vi "BASE_Reporting.vi"(8 "error in (no error)":errorcluster) -> (0 "error out":errorcluster)   [LabVIEW 2017]
uses:
  <vilib>/Utility/miscctls.llb/LVRangeTypeDef.ctl
  <vilib>/Utility/miscctls.llb/LVRowAndColumnTypeDef.ctl
  <vilib>/Utility/miscctls.llb/LVRowAndColumnUnsignedTypeDef.ctl
  <vilib>/addons/database/Connection.llb/DB Tools Open Connec (Path).vi
  <vilib>/Utility/file.llb/Write Delimited Spreadsheet (string).vi
  <vilib>/addons/database/NI_Database_API.lvlib
panel:
  in  "Horizontal Slider Control":dbl(slide)=1.0 scale=0.0..19.0
  in  "Vertical Slider Control":dbl(slide)=1.0
  out "From Date":string
  out "appended path":path
  in  "SELECT FILTER":string(combo)="PART_NO"
  in  "Export to Excel":bool
  out "DESCRIPTION":string
  out "Data History Table":string[][](table)
  in  "TO DATE":timestamp format="%<%d/%m/%Y>T"
  in  "FROM DATE":timestamp format="%<%d/%m/%Y>T"
  in  "Back":bool
  in  "Show Report":bool
  # "BARCODE VERIFICATION SYSTEM REPORTS"
  # "Data History Table"
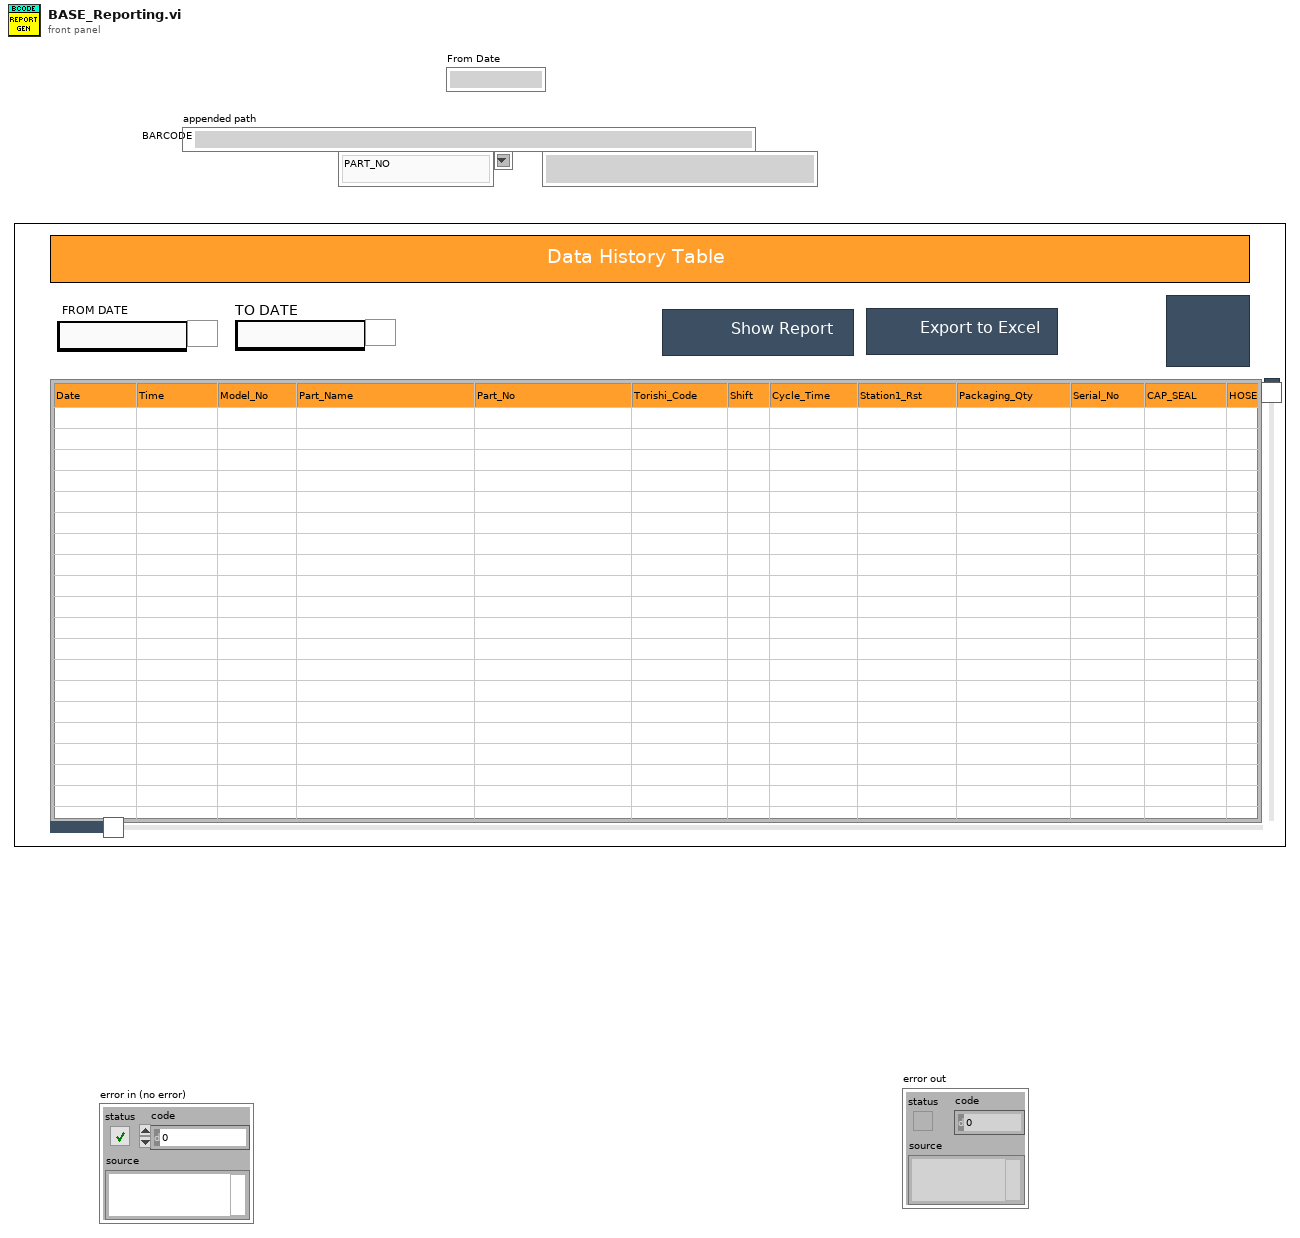
[diagram p1: front panel]
types:
  T1 = typedef "NI_Database_API.lvlib/Conn ObjectReference.ctl" = refnum<k1>
  T2 = typedef "LVRangeTypeDef.ctl" = cluster{"Minimum":dbl, "Maximum":dbl, "Increment":dbl, "Minor Increment":dbl, "Start":dbl}
  T3 = typedef "LVRowAndColumnTypeDef.ctl" = cluster{"Row":i32, "Column":i32}
  T4 = typedef "LVRowAndColumnUnsignedTypeDef.ctl" = cluster{"Row":u32, "Column":u32}
  T5 = enum32{"Invalid", "Standard", "Closed", "Hidden", "Minimized", "Maximized"}
  T6 = enum32{"invalid app kind", "Development System", "Run Time System", "Student Edition", "Embedded LabVIEW", "Evaluation", "Custom"}
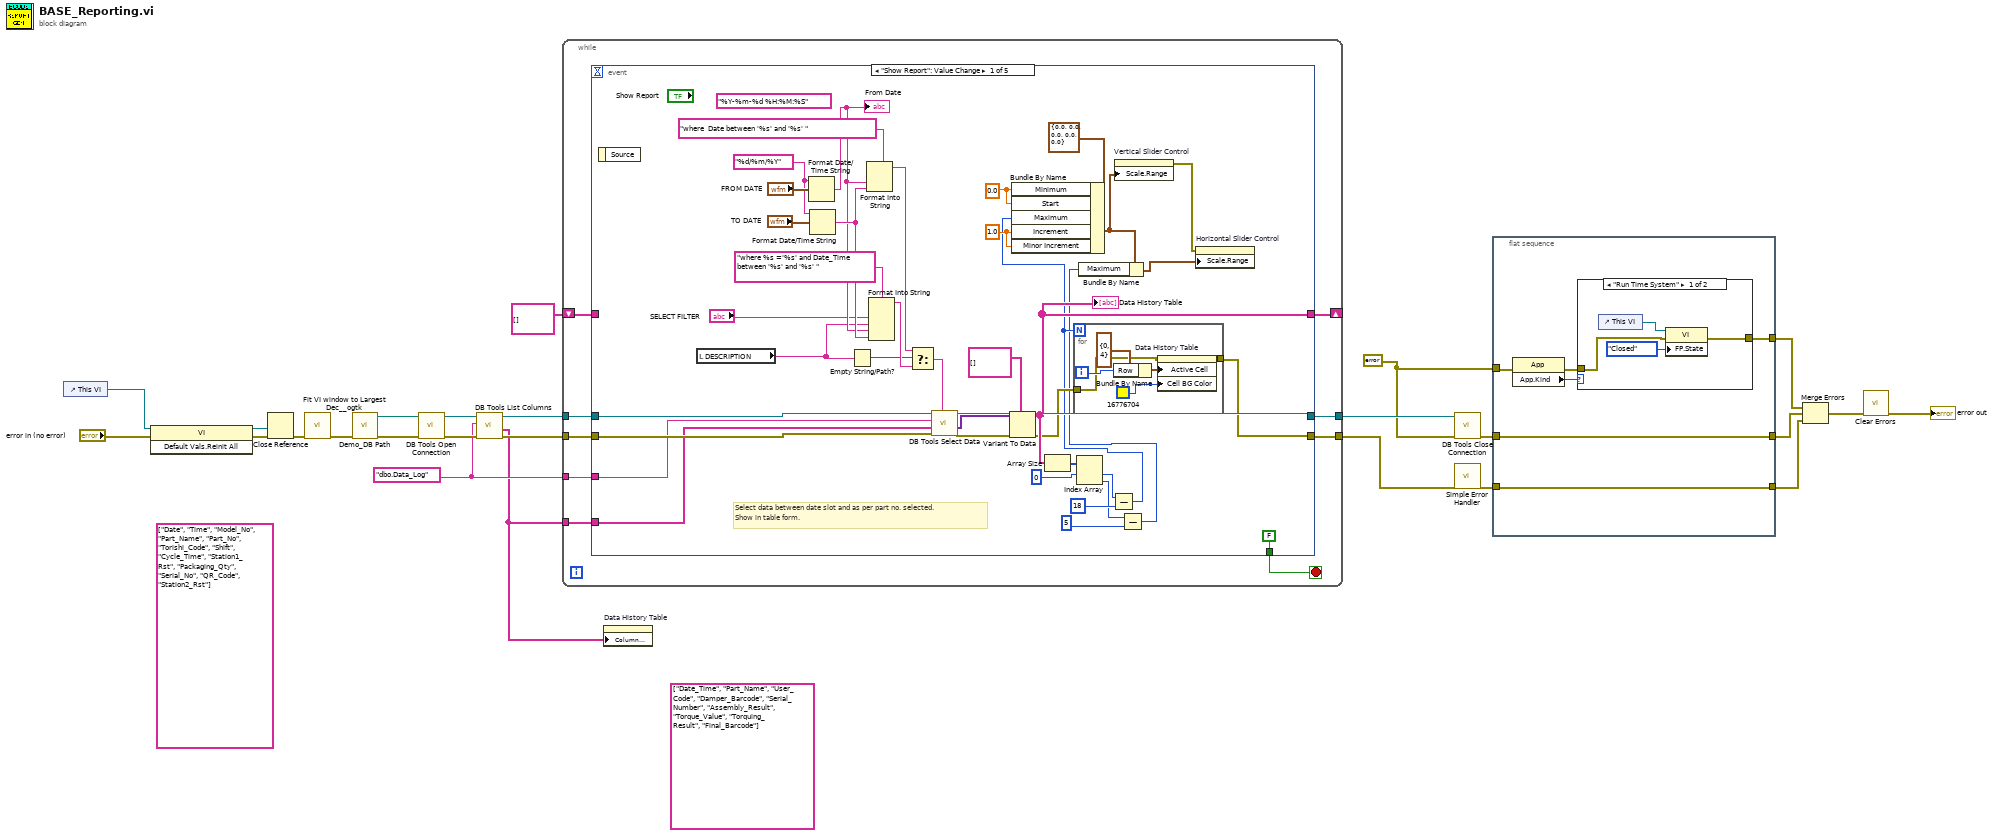
[diagram p0: block diagram]
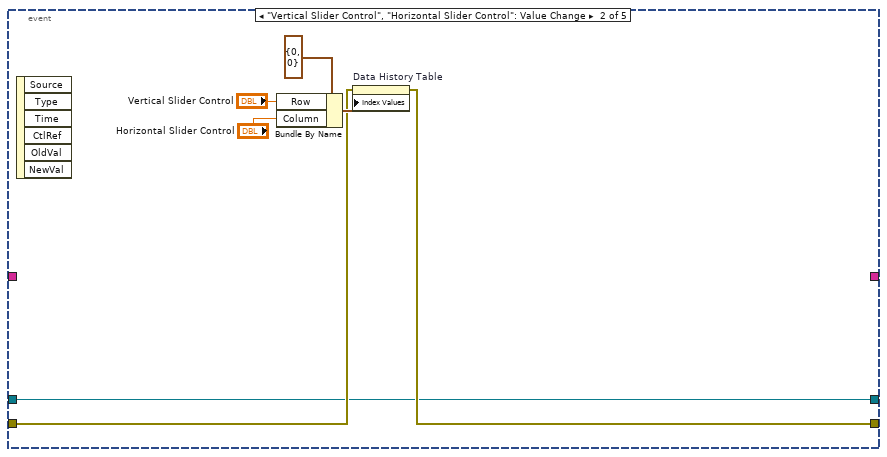
[diagram p3: hidden frame]
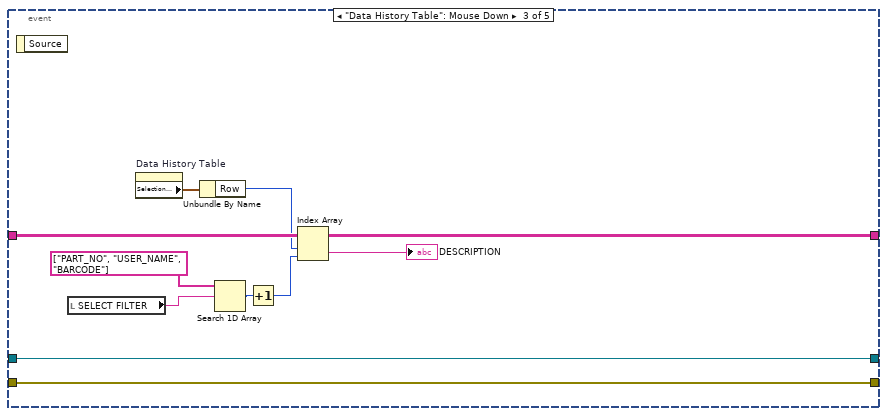
[diagram p4: hidden frame]
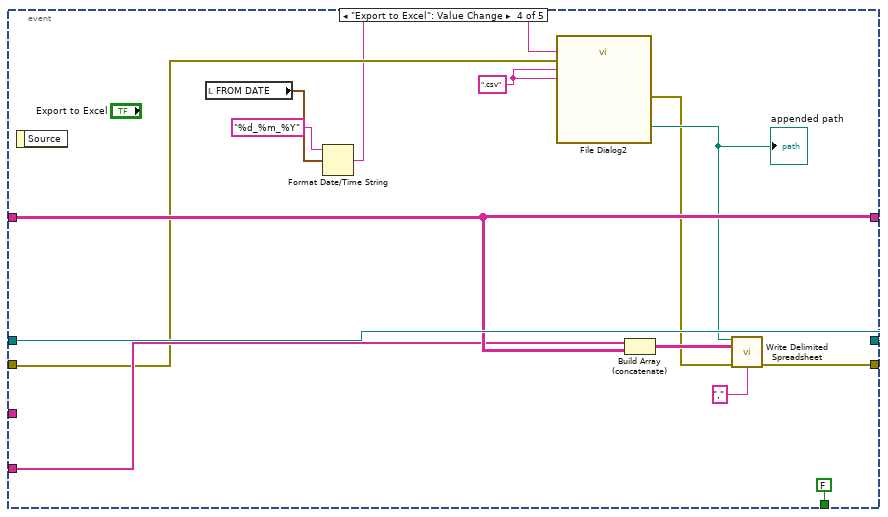
[diagram p5: hidden frame]
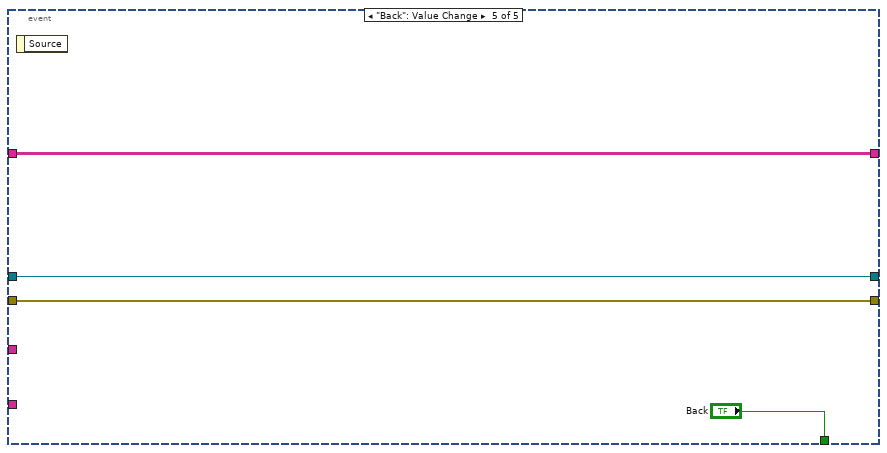
[diagram p6: hidden frame]
diagram:
  (unwired) string[] ["Date", "Time", "Model_No", "Part_Name", "Part_No", "Torishi_Code", "Shift", "Cycle_Time", "Station1_Rst", "Packaging_Qty", "Serial_No", "QR_Code", "Station2_Rst"] ("columns 2")
  w2 = "dbo.Data_Log" ("table")
  (unwired) string[] ["Date_Time", "Part_Name", "User_Code", "Damper_Barcode", "Serial_Number", "Assembly_Result", "Torque_Value", "Torquing_Result", "Final_Barcode"]
  w20 = errorcluster {"status"=FALSE, "code"=0, "source"=""} ("error in (no error)")
  n1 = control-ref of="This VI"() -> (w14:refnum<vi>)
  n2 = invoke class="VI" method="Default Vals.Reinit All"(reference=w14, error in="error in (no error)") -> (reference out=w12:refnum<vi>, error out=w11:errorcluster)  [unwired: 1 in, 1 out]
  n3 = Close Reference(reference=w12, error in (no error)=w11) -> (error out=w10:errorcluster)
  n4 = call <userlib>:"Fit VI window to Largest Dec__ogtk.vi"("error in (no error)"=w10) -> ("error out"=w3:errorcluster)  [unwired: 5 in, 1 out]
  n5 = call "Demo_DB Path.vi"("error in"=w3) -> ("error out"=w9:errorcluster, "DB Path"=w8:path)  [unwired: 9 in]
  n6 = call-poly <vilib>:"DB Tools Open Connection.vi"("error in (no error)"=w9, "connection information"=w8) -> ("error out"=w7:errorcluster, "connection reference"=w5:T1)  [unwired: 6 in]
  n7 = call <vilib>:"DB Tools List Columns.vi"("error in (no error)"=w7, "table"=w2, "connection reference"=w5) -> ("error out"=w6:errorcluster, "columns"=w1:string[], "connection reference out"=w4:T1)  [unwired: 1 in, 1 out]
  n8 = while {
    tunnel: w1 -> [w30]
    tunnel: w2 -> [w29]
    tunnel: w4 -> [w34]
    tunnel: [w31] -> w25
    tunnel: w6 -> [w33]
    tunnel: [w32] -> w23
    shift-right: [w27] -> _
    shift-left: string[][] [] -> [w26]
    stop <- w28 stop-if-true
    n9 = event shown="[0] \"Show Report\": Value Change" {
      selector: _ -> [_ _ _ _ _]
      dyn-events: _ -> [_ _ _ _ _]
      timeout: _ -> [_ _ _ _ _]
      tunnel: w34 -> [w73 w81 w93 w110 w113]
      tunnel: w33 -> [w72 w83 w92 w101 w112]
      tunnel: [w47 w82 w92 w105 w112] -> w32
      tunnel: [w71 w81 w93 w110 w113] -> w31
      tunnel: w30 -> [w70 _ _ w106 _]
      tunnel: w29 -> [w69 _ _ _ _]
      tunnel: [FALSE ("Back") _ _ FALSE ("Back") "Back"] -> w28
      tunnel: [w51 _ w96 w107 w111] -> w27
      tunnel: w26 -> [_ _ w96 w107 w111]
      event "Show Report": Value Change {
        w35 = 0.0 ("Start")
        w45 = 1.0 ("Increment")
        (unwired) "%Y-%m-%d %H:%M:%S"
        w58 = "%d/%m/%Y"
        # "Select data between date slot and as per part no. selected.\nShow in table form."
        n10 = event-data() -> ()  [unwired: 1 in, 1 out]
        n11 = local read "DESCRIPTION"() -> (w52:string)
        n12 = Format Date/Time String(time format string (%c)=w58, seconds (now)="FROM DATE") -> (date/time string=w54:string)  [unwired: 1 in]
        "From Date" <- w54
        n13 = Format Date/Time String(time format string (%c)=w58, seconds (now)="TO DATE") -> (date/time string=w55:string)  [unwired: 1 in]
        n14 = Empty String/Path?(string/path=w52) -> (empty?=w56:bool)
        n15 = Format Into String(format string="where  Date between '%s' and '%s' ", w54, w55) -> (resulting string=w63:string)  [unwired: 2 in, 1 out]
        n16 = Format Into String(format string="where %s ='%s' and Date_Time between '%s' and '%s' ", "SELECT FILTER", w52, w54, w55) -> (resulting string=w64:string)  [unwired: 2 in, 1 out]
        n17 = Select(t=w63, s=w56, f=w64) -> (s? t:f=w57:string)
        n18 = call <vilib>:"DB Tools Select Data.vi"("condition"=w57, "error in (no error)"=w72, "columns"=w70, "table"=w69, "connection reference"=w73) -> ("error out"=w65:errorcluster, "data"=w68:variant[][], "connection reference out"=w71:T1)  [unwired: 1 in]
        n19 = Variant To Data(error in=w65, type=string[][] [], Variant=w68) -> (data=w51:string[][], error out=w48:errorcluster)
        "Data History Table" <- w51
        n20 = Array Size(array=w51) -> (size(s)=w50:i32[])
        n21 = Index Array(array=w50, index #1=0 ("index")) -> (element #1=w40:i32, element #2=w37:i32)  [unwired: 1 in]
        n22 = Subtract(x=w40, y=18) -> (x-y=w39:i32)
        n23 = Bundle By Name(cluster=T2 {"Minimum"=0.0, "Maximum"=0.0, "Increment"=0.0, "Minor Increment"=0.0, "Start"=0.0} ("Scale.Range"), "Minimum"=w35, "Start"=w35, "Maximum"=w39, "Increment"=w45, "Minor Increment"=w45) -> (w44:T2)
        n24 = for {
          N: w39 -> [_]
          tunnel: w48 -> [w75]
          tunnel: [w74] -> w47
          i -> [w77]
          n25 = Bundle By Name(cluster=T3 {"Row"=0, "Column"=4} ("Active Cell:Active Cell"), "Row"=w77) -> (w78:T3)
          n26 = property on="Data History Table" class="Tbl (strict)"(error in=w75, "Active Cell"=w78, "Cell BG Color"=u32 16776704) -> (error out=w74:errorcluster)  [unwired: 1 in, 1 out]
        }
        n27 = property on="Vertical Slider Control" class="Slide (strict)"("Scale.Range"=w44) -> (error out=w42:errorcluster)  [unwired: 2 in, 1 out]
        n28 = Subtract(x=w37, y=5) -> (x-y=w38:i32)
        n29 = Bundle By Name(cluster=w44, "Maximum"=w38) -> (w43:T2)
        n30 = property on="Horizontal Slider Control" class="Slide (strict)"(error in=w42, "Scale.Range"=w43) -> ()  [unwired: 1 in, 2 out]
      }
      event "Vertical Slider Control", "Horizontal Slider Control": Value Change {
        n31 = event-data() -> ()  [unwired: 1 in, 6 out]
        n32 = Bundle By Name(cluster=T4 {"Row"=0, "Column"=0} ("Index Values"), "Row"="Vertical Slider Control", "Column"="Horizontal Slider Control") -> (w86:T4)
        n33 = property on="Data History Table" class="Tbl (strict)"(error in=w83, "Index Values"=w86) -> (error out=w82:errorcluster)  [unwired: 1 in, 1 out]
      }
      event "Data History Table": Mouse Down {
        n34 = event-data() -> ()  [unwired: 1 in, 1 out]
        n35 = local read "SELECT FILTER"() -> (w89:string)
        n36 = property on="Data History Table" class="Tbl (strict)"() -> ("Selection Start"=w95:T3)  [unwired: 2 in, 2 out]
        n37 = Unbundle By Name(w95) -> ("Row"=w94:i32)
        n38 = Search 1D Array(1D array=string[] ["PART_NO", "USER_NAME", "BARCODE"], element=w89) -> (index of element=w88:i32)  [unwired: 1 in]
        n39 = Increment(x=w88) -> (x+1=w87:i32)
        n40 = Index Array(array=w96, index (row)=w94, index (col)=w87) -> (element=→"DESCRIPTION":string)
      }
      event "Export to Excel": Value Change {
        w104 = ".csv" ("pattern label")
        n41 = event-data() -> ()  [unwired: 1 in, 1 out]
        n42 = local read "FROM DATE"() -> (w99:timestamp)
        n43 = Format Date/Time String(time format string (%c)="%d_%m_%Y", seconds (now)=w99) -> (date/time string=w98:string)  [unwired: 1 in]
        n44 = call "File Dialog2"("default name"=w98, "error in"=w101, "pattern (all files)"=w104, "pattern label"=w104) -> ("selected path"=w103:path, "error out"=w102:errorcluster)  [unwired: 8 in, 2 out]
        "appended path" <- w103
        n45 = Build Array (concatenate)(w106, w107) -> (w108:string[][])
        n46 = call-poly <vilib>:"Write Delimited Spreadsheet.vi"("file path (dialog if empty)"=w103, "2D data"=w108, "error in (no error)"=w102, "delimiter (\\t)"="," ("delimiter (\\t)")) -> ("error out"=w105:errorcluster)  [unwired: 10 in, 1 out]
      }
      event "Back": Value Change {
        n47 = event-data() -> ()  [unwired: 1 in, 1 out]
      }
    }
  }
  n48 = property on="Data History Table" class="Tbl (strict)"("Column Headers[]"=w1) -> ()  [unwired: 2 in, 2 out]
  n49 = call <vilib>:"DB Tools Close Connection.vi"("error in (no error)"=w20, "connection reference"=w25) -> ("error out"=w18:errorcluster)  [unwired: 5 in]
  n50 = call <vilib>:"Simple Error Handler.vi"("error in (no error)"=w23) -> ("error out"=w16:errorcluster)  [unwired: 4 in, 4 out]
  n51 = flat-sequence {
    tunnel: [w118] -> w21
    tunnel: w20 -> [w117]
    tunnel: [w116] -> w19
    tunnel: w18 -> [w116]
    tunnel: [w115] -> w17
    tunnel: w16 -> [w115]
    frame #0 {
      n52 = property class="App"(error in=w117) -> (error out=w119:errorcluster, "App.Kind"=w120:T6)  [unwired: 1 in, 1 out]
      n53 = case shown="\"Run Time System\"" w120 {
        tunnel: w119 -> [w122 w125]
        tunnel: [w121 w125] -> w118
        frame "Run Time System" {
          n54 = control-ref of="This VI"() -> (w124:refnum<vi>)
          n55 = property class="VI"(reference=w124, error in=w122, "FP.State"=T5."Closed" ("Front Panel Window:State")) -> (error out=w121:errorcluster)  [unwired: 1 out]
        }
        frame "Development System", Default {
        }
      }
    }
  }
  n56 = Merge Errors(w21, w19, w17) -> (w22:errorcluster)
  n57 = call <vilib>:"Clear Errors.vi"("error in (no error)"=w22) -> ("error out"=→"error out":errorcluster)  [unwired: 5 in, 1 out]
